vi "Auto Shifting.vi"() -> ()   [LabVIEW 2018]
uses:
  Sensor Readings.vi
  Robot States.vi
panel:
  in  "Time Above Speed (ms)":u32
  in  "Switch to Low Gear (ft/s)":dbl
  in  "Switch to High Gear (ft/s)":dbl
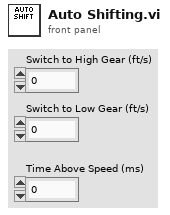
[diagram p1: front panel]
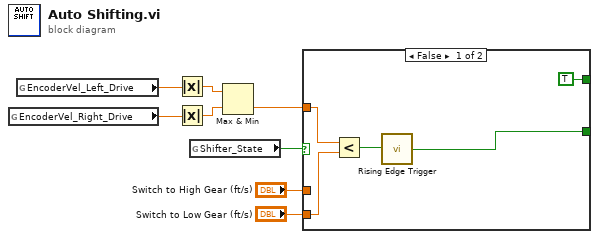
[diagram p0: block diagram]
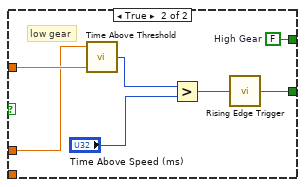
[diagram p2: hidden frame]
diagram:
  n1 = global read "Sensor Readings.vi" "EncoderVel_Right_Drive"() -> (w7:dbl)
  n2 = global read "Sensor Readings.vi" "EncoderVel_Left_Drive"() -> (w8:dbl)
  n3 = Absolute Value(x=w8) -> (abs(x)=w5:dbl)
  n4 = Absolute Value(x=w7) -> (abs(x)=w6:dbl)
  n5 = global read "Robot States.vi" "Shifter_State"() -> (w2:bool)
  n6 = Max & Min(x=w5, y=w6) -> (min(x,y)=w4:dbl)  [unwired: 1 out]
  n7 = case shown="False" w2 {
    tunnel: w4 -> [w13 w20]
    tunnel: "Switch to High Gear (ft/s)" -> [_ w19]
    tunnel: [w10 w15] -> _
    tunnel: [TRUE ("High Gear") w14] -> _
    tunnel: "Switch to Low Gear (ft/s)" -> [w12 _]
    frame False {
      n8 = Less?(x=w13, y=w12) -> (x < y?=w11:bool)
      n9 = call "Rising Edge Trigger.vi"("Raw Signal"=w11) -> ("Trigger"=w10:bool)
    }
    frame True {
      w14 = FALSE  # High Gear
      # "low gear"
      n10 = call "Time Above Threshold.vi"("Current Value"=w20, "Threshold"=w19) -> ("Time Above"=w18:u32)  [unwired: 3 in]
      n11 = Greater?(x=w18, y="Time Above Speed (ms)") -> (0:w16:bool)
      n12 = call "Rising Edge Trigger.vi"("Raw Signal"=w16) -> ("Trigger"=w15:bool)
    }
  }
